vi "Add JSON Schema.vi"(8 "error in (no error)":errorcluster, 9 "Object Name":string, 10 "Object":variant, 11 "JSON Schema in":string) -> (0 "error out":errorcluster, 3 "JSON Schema out":string)   [LabVIEW 2019, in "JSON-Schema.lvlib"]
uses:
  JSON-Schema.lvlib
  <vilib>/JDP Science/JSONtext/JSONtext.lvlib
  <vilib>/Utility/Data Type/NI_Data Type.lvlib
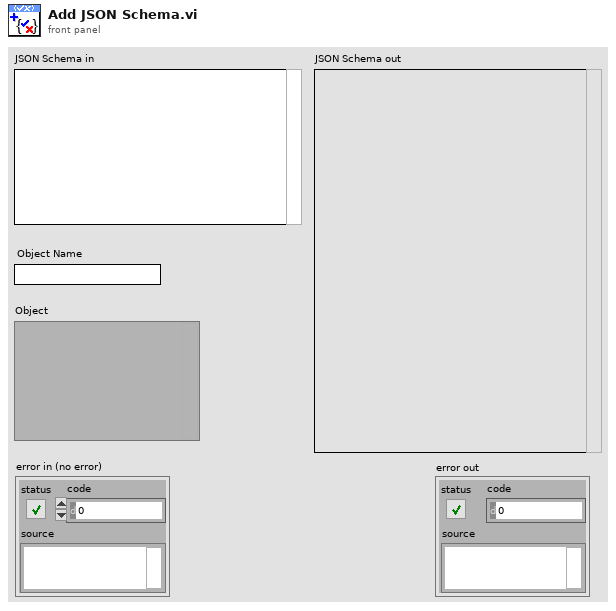
[diagram p1: front panel]
types:
  T1 = enum32{"Bad", "Idle", "Run top level", "Running"}
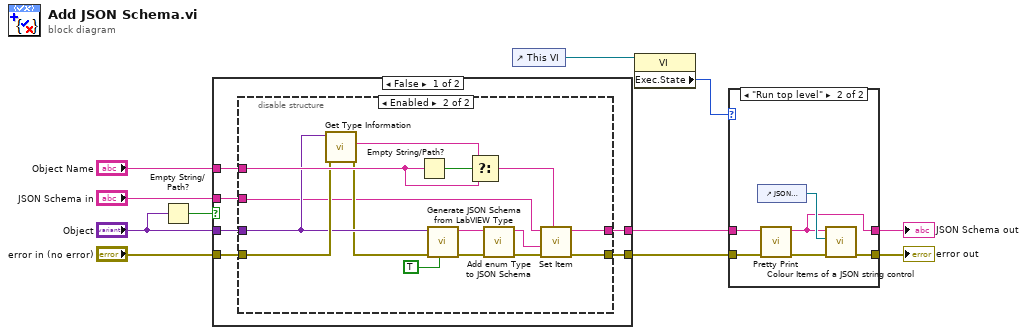
[diagram p0: block diagram]
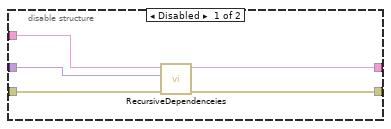
[diagram p2: hidden frame]
diagram:
  n1 = Empty String/Path?(string/path="Object") -> (empty?=w1:bool)
  n2 = case shown="False" w1 {
    tunnel: "error in (no error)" -> [w17 w39]
    tunnel: [w16 w38] -> w7
    tunnel: [w15 w39] -> w6
    tunnel: "Object Name" -> [w14 _]
    tunnel: "JSON Schema in" -> [w13 w38]
    tunnel: "Object" -> [w12 _]
    frame False {
      n3 = disable-structure shown="Enabled" {
        disable-tunnel: w12 -> [w22 w25]
        disable-tunnel: w17 -> [w21 w26]
        disable-tunnel: w13 -> [w20 w23]
        disable-tunnel: [w19 w33] -> w16
        disable-tunnel: [w18 w32] -> w15
        disable-tunnel: w14 -> [_ w28]
        frame Disabled {
          n4 = call "RecursiveDependenceies.vi"("error in (no error)"=w21, "Object"=w22, "JSON Schema in"=w20) -> ("error out"=w18:errorcluster, "JSON Schema out"=w19:string)  [unwired: 7 in]
        }
        frame Enabled {
          n5 = call <vilib>:"Get Type Information.vi"("error in (no error)"=w26, "variant"=w25) -> ("error out"=w24:errorcluster, "name"=w29:string)  [unwired: 5 in, 3 out]
          n6 = Empty String/Path?(string/path=w28) -> (empty?=w31:bool)
          n7 = call <vilib>:"Generate JSON Schema from LabVIEW Type.vi"("Strict Clusters"=TRUE, "error in (no error)"=w24, "Variant"=w25) -> ("error out"=w37:errorcluster, "JSON Schema"=w36:string)  [unwired: 7 in]
          n8 = Select(t=w29, s=w31, f=w28) -> (s? t:f=w30:string)
          n9 = call "Add enum Type to JSON Schema.vi"("error in (no error)"=w37, "JSON Schema in"=w36) -> ("error out"=w35:errorcluster, "JSON Schema out"=w34:string)  [unwired: 8 in]
          n10 = call <vilib>:"Set Item.vi"("$Path or Item Name"=w30, "error in (no error)"=w35, "JSON to Insert"=w34, "JSON"=w23) -> ("error out"=w32:errorcluster, "<JSON>"=w33:string)  [unwired: 4 in, 1 out]
        }
      }
    }
    frame True {
    }
  }
  n11 = control-ref of="This VI"() -> (w11:refnum<vi>)
  n12 = property class="VI"(reference=w11) -> ("Exec.State"=w4:T1)  [unwired: 1 in, 2 out]
  n13 = case shown="\"Run top level\"" w4 {
    tunnel: w7 -> [w40 w47]
    tunnel: w6 -> [w41 w46]
    tunnel: [w41 w44] -> w10
    tunnel: [w40 w42] -> w9
    frame Default {
    }
    frame "Run top level" {
      n14 = control-ref of="JSON Schema out"() -> (w43:refnum<vi>)
      n15 = call <vilib>:"Pretty Print.vi"("error in (no error)"=w46, "JSON"=w47) -> ("error out"=w45:errorcluster, "<JSON>"=w42:string)  [unwired: 7 in, 1 out]
      n16 = call <vilib>:"Colour Items of a JSON string control.vi"("error in (no error)"=w45, "String Control"=w43, "JSON"=w42) -> ("error out"=w44:errorcluster)  [unwired: 8 in]
    }
  }
  "JSON Schema out" <- w9
  "error out" <- w10
